vi "Measure [MSR] Core.vi"(8 "error in (no error)":errorcluster, 9 "measurement type (voltage)":i32(ring)=1 items=["Voltage"=1, "Current"=0], 10 "channel name (\"CHANNEL1\")":string="CHANNEL1", 11 "IVI_DCPwr in":refnum<class "IVI_DCPwr.lvclass">) -> (0 "error out":errorcluster, 2 "measurement":dbl format="%^.2e", 3 "IVI_DCPwr out":refnum<class "IVI_DCPwr.lvclass">)   [LabVIEW 2015, in "IVI_DCPwr.lvlib" / "IVI_DCPwr.lvclass"]
doc: "This VI takes a single measurement on the channel you specify.\n\nNotes:\n\n(1) This VI is part of the IviDCPwrMeasure [MSR] extension group."
uses:
  IVI_DCPwr.lvclass
  IVI_DCPwr.lvclass/IVI_DCPwr.ctl
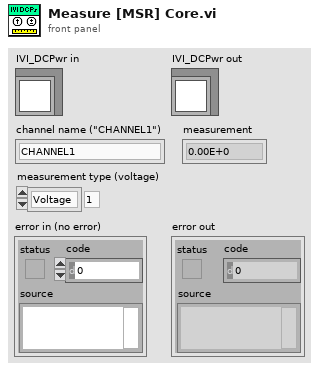
[diagram p1: front panel]
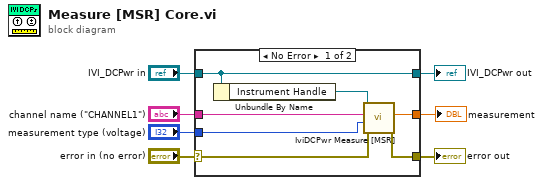
[diagram p0: block diagram]
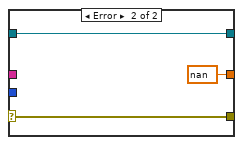
[diagram p2: hidden frame]
diagram:
  n1 = case shown="No Error" "error in (no error)" {
    selector: "error in (no error)" -> [w12 w17]
    tunnel: [w11 w17] -> w6
    tunnel: [w14 w16] -> w4
    tunnel: "IVI_DCPwr in" -> [w14 w16]
    tunnel: "channel name (\"CHANNEL1\")" -> [w10 _]
    tunnel: "measurement type (voltage)" -> [w9 _]
    tunnel: [w8 nan ("measurement")] -> w1
    frame No Error {
      n2 = Unbundle By Name(w14) -> ("Instrument Handle"=w13:refnum<k15>)
      n3 = call <vilib>:"IviDCPwr Measure [MSR].vi"("error in (no error)"=w12, "measurement type (voltage)"=w9, "channel name (\"CHANNEL1\")"=w10, "instrument handle"=w13) -> ("error out"=w11:errorcluster, "measurement"=w8:dbl)  [unwired: 5 in, 1 out]
    }
    frame Error {
    }
  }
  "error out" <- w6
  "IVI_DCPwr out" <- w4
  "measurement" <- w1
